vi "Check_and_rewrite_file.vi"(0 "Filename":path, 7 "Present Channels only":bool, 9 "Present Channels":string[](array[string]), 11 "Start of read offset (chars.: 0)":i32) -> (4 "exists?":bool, 6 "Merged Channels":string[](array[string]), 8 "Start of data (bytes)":i32, 10 "No of bytes/row (approx)":i32, 14 "Current file size (bytes)":i32, 15 "Merged?":bool)   [LabVIEW 2014]
uses:
  Anemometry/Anemometry Sub Vis/Globals/Constants_global.vi
panel:
  in  "stop":bool
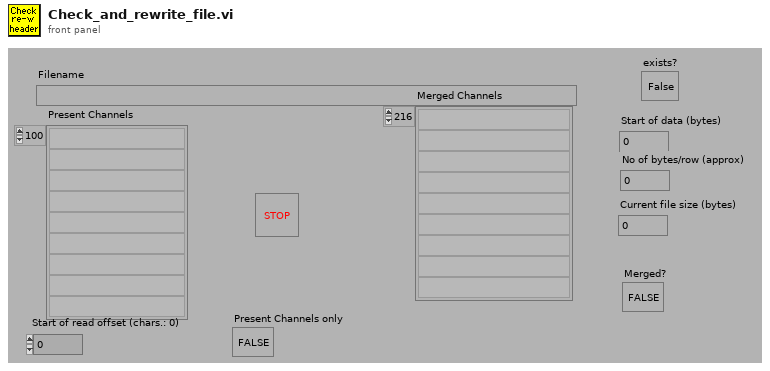
[diagram p1: front panel]
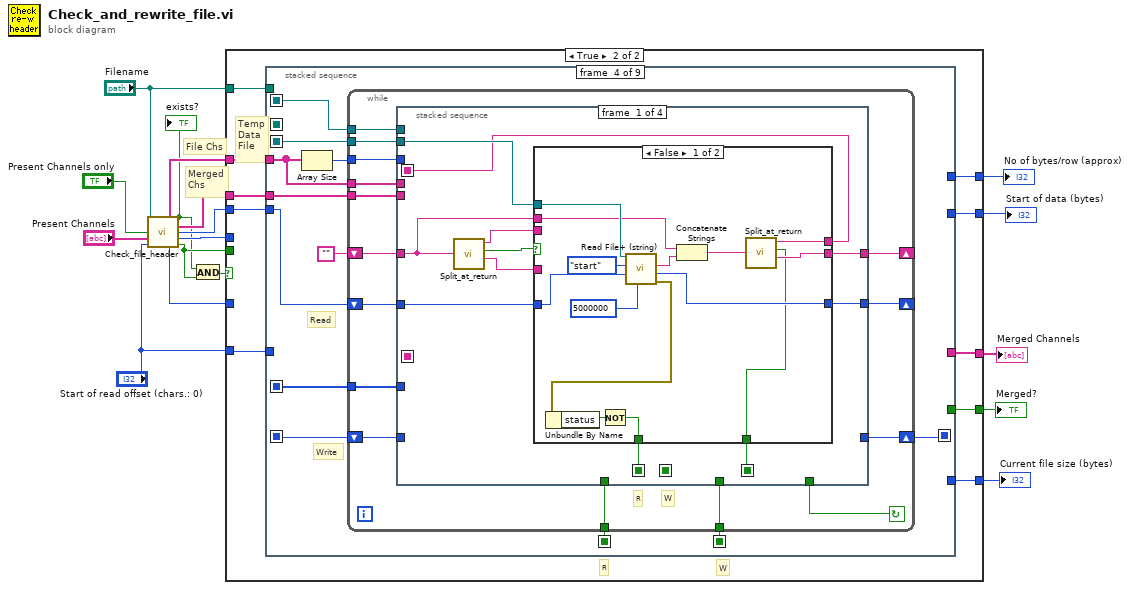
[diagram p0: block diagram]
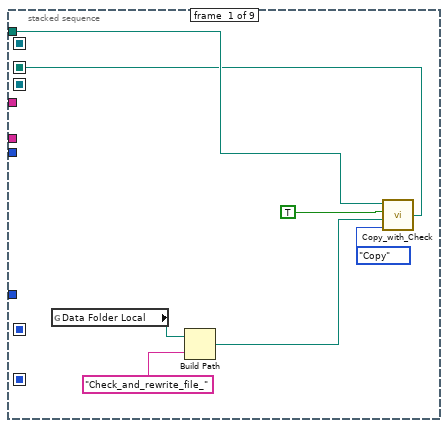
[diagram p3: hidden frame]
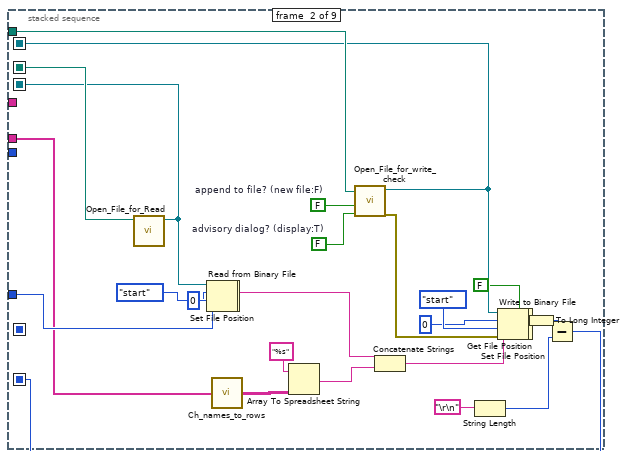
[diagram p4: hidden frame]
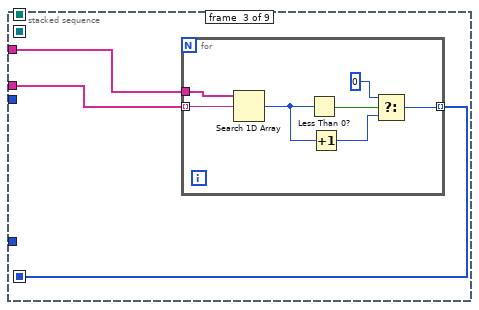
[diagram p5: hidden frame]
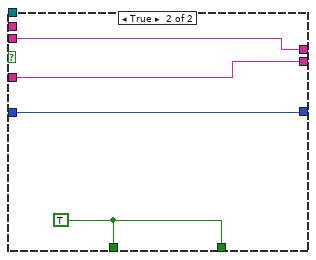
[diagram p6: hidden frame]
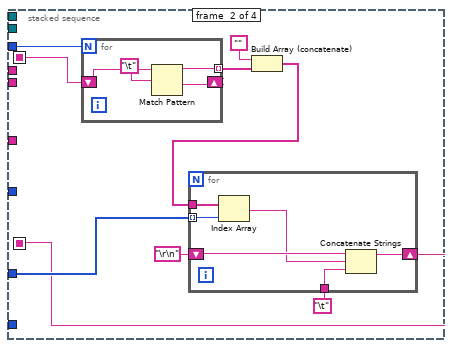
[diagram p7: hidden frame]
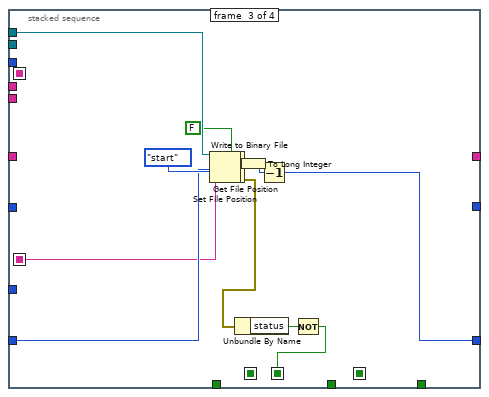
[diagram p8: hidden frame]
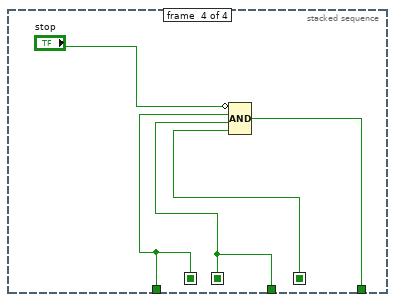
[diagram p9: hidden frame]
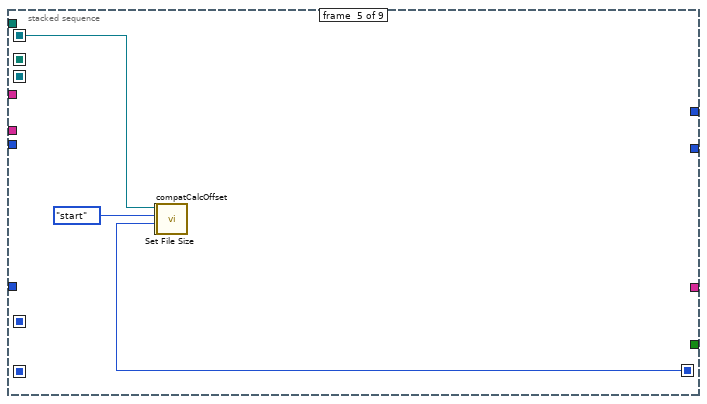
[diagram p10: hidden frame]
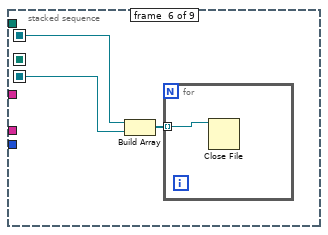
[diagram p11: hidden frame]
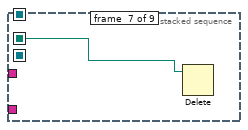
[diagram p12: hidden frame]
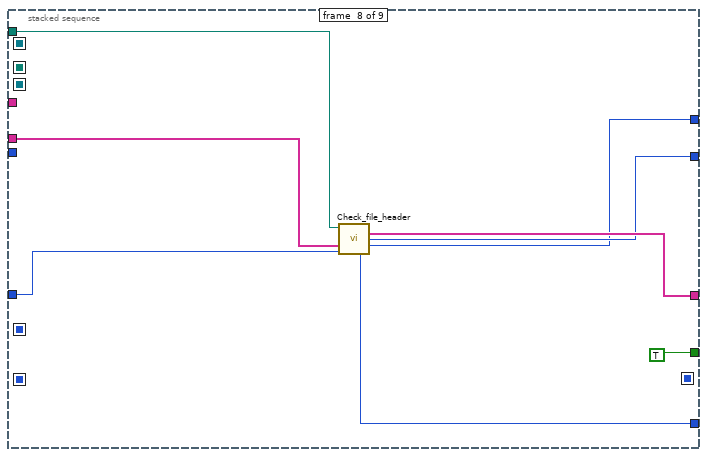
[diagram p13: hidden frame]
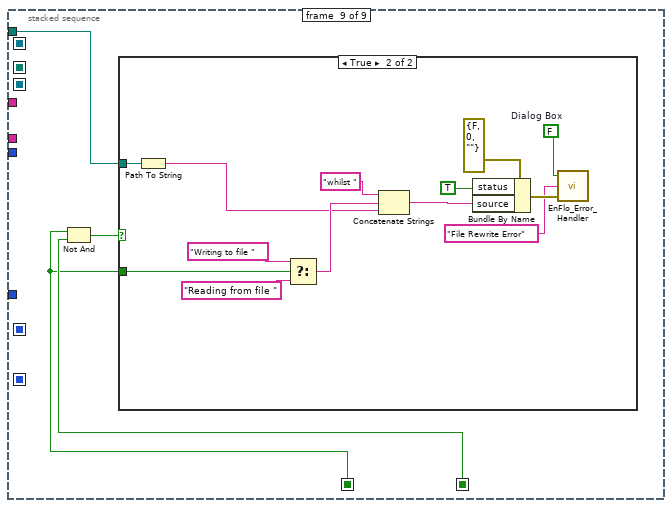
[diagram p14: hidden frame]
diagram:
  # "Merged\nChs"
  # "File Chs"
  n1 = call "Check_file_header.vi"("Filename"="Filename", "Present Channels only"="Present Channels only", "Present Channels"="Present Channels", "Start of read offset (chars.: 0)"="Start of read offset (chars.: 0)") -> ("File Channels"=w5:string[], "exists?"=w4:bool, "Merged Channels"=w11:string[], "Start of data (bytes)"=w10:i32, "No of bytes/row (approx)"=w9:i32, "Current file size (bytes)"=w8:i32, "Merged?"=w12:bool)  [unwired: 5 out]
  "exists?" <- w4
  n2 = And(x=w4, y=w12) -> (x .and. y?=w1:bool)
  n3 = case shown="True" w1 {
    tunnel: [w21 w30] -> w17
    tunnel: [w22 w29] -> w16
    tunnel: [w19 w27] -> w15
    tunnel: [w20 w28] -> w14
    tunnel: [w18 w26] -> w13
    tunnel: w12 -> [w22 _]
    tunnel: w11 -> [w21 w31]
    tunnel: w10 -> [w20 w24]
    tunnel: w9 -> [w19 _]
    tunnel: w8 -> [w18 _]
    tunnel: "Start of read offset (chars.: 0)" -> [_ w25]
    tunnel: w5 -> [_ w23]
    tunnel: "Filename" -> [_ w32]
    frame False {
    }
    frame True {
      # "W"
      # "R"
      # "Temp\nData\nFile"
      n4 = stacked-sequence {
        seq-local: [w34 _ _ _ _ _ _ _ _] -> [_ w66 _ _ _ _ w185 _ _]
        seq-local: [_ w48 _ _ _ _ _ _ _] -> [_ _ _ w90 _ w182 _ _ _]
        seq-local: [_ w65 _ _ _ _ _ _ _] -> [_ _ _ w84 w180 w183 _ _ _]
        seq-local: [_ w58 _ _ _ _ _ _ _] -> [_ _ _ w88 _ _ _ _ _]
        seq-local: [_ _ _ w83 _ _ _ _ _] -> [_ _ _ _ _ _ _ _ w195]
        seq-local: [_ _ _ w82 _ _ _ _ _] -> [_ _ _ _ _ _ _ _ w197]
        seq-local: [_ _ w70 _ _ _ _ _ _] -> [_ _ _ w81 _ _ _ _ _]
        seq-local: [_ _ _ w80 _ _ _ _ _] -> [_ _ _ _ w179 _ _ _ _]
        tunnel: w32 -> [w36 w67 _ _ _ _ _ w192 w194]
        tunnel: w31 -> [_ w50 w72 w85 _ _ _ w193 _]
        tunnel: [_ _ _ _ _ _ _ w191 _] -> w30
        tunnel: [_ _ _ _ _ _ _ TRUE _] -> w29
        tunnel: [_ _ _ _ _ _ _ w189 _] -> w28
        tunnel: [_ _ _ _ _ _ _ w188 _] -> w27
        tunnel: [_ _ _ _ _ _ _ w187 _] -> w26
        tunnel: w25 -> [_ w52 _ _ _ _ _ w186 _]
        tunnel: w24 -> [_ _ _ w89 _ _ _ _ _]
        tunnel: w23 -> [_ _ w71 w86 _ _ _ _ _]
        frame #0 {
          n5 = global read "Constants_global.vi" "Data Folder Local"() -> (w39:path)
          n6 = Build Path(base path=w39, name or relative path="Check_and_rewrite_file_") -> (appended path=w35:path)
          n7 = call "Copy_with_Check.vi"("Mode"=enum16{"Move", "Copy"}."Copy", "Target Path"=w35, "Variable Target?"=TRUE, "Source Path"=w36) -> ("Pathname Out"=w34:path)
        }
        frame #1 {
          w68 = FALSE  # advisory dialog? (display:T)
          w69 = FALSE  # append to file? (new file:F)
          n8 = call "Open_File_for_Read.vi"("file path"=w66) -> ("refnum"=w48:refnum<file>)  [unwired: 1 in, 9 out]
          n9 = Set File Position(offset (in bytes) (0)=0 ("pos offset (0)"), refnum=w48, from (0:start)=enum16{"start", "end", "current"}."start" ("pos mode (rel. to current:2)")) -> (refnum out=w47:refnum<file>, error out=w46:errorcluster)  [unwired: 1 in]
          n10 = Read from Binary File(8:w46, 10:w52, 11:w47) -> (2:w54:string)  [unwired: 6 out]
          n11 = call "Ch_names_to_rows.vi"("Channel Names"=w50) -> ("3 Row names"=w49:string[][])
          n12 = Array To Spreadsheet String(array=w49, 3:"%s" ("format string")) -> (spreadsheet string=w55:string)  [unwired: 1 out]
          n13 = call "Open_File_for_write_check.vi"("advisory dialog? (display:T)"=w68, "append to file? (new file:F)"=w69, "file path"=w67) -> ("error out"=w62:errorcluster, "refnum"=w65:refnum<file>)  [unwired: 7 out]
          n14 = Concatenate Strings(w54, w55) -> (w53:string)
          n15 = String Length(string="\r\n") -> (length=w59:i32)
          n16 = Set File Position(offset (in bytes) (0)=0 ("pos offset (0)"), refnum=w65, from (0:start)=enum16{"start", "end", "current"}."start" ("pos mode (0:2)"), error in=w62) -> (refnum out=w45:refnum<file>, error out=w44:errorcluster)
          n17 = Write to Binary File(file (use dialog)=w45, data=w53, error in=w44, 5:FALSE ("prepend array or string size? (T)")) -> (refnum out=w43:refnum<file>, error out=w42:errorcluster)  [unwired: 3 out]
          n18 = Get File Position(4:w42, 7:w43) -> (2:w41:i64)  [unwired: 2 out]
          n19 = To Long Integer(number=w41) -> (32bit integer=w60:i32)
          n20 = Subtract(x=w60, y=w59) -> (x-y=w58:i32)
        }
        frame #2 {
          n21 = for {
            tunnel: w71 -> [w79]
            tunnel: w72 -> [w78] mode=indexing
            tunnel: [w73] -> w70 mode=indexing
            n22 = Search 1D Array(1D array=w79, element=w78) -> (index of element=w76:i32)  [unwired: 1 out]
            n23 = Less Than 0?(x=w76) -> (x < 0?=w77:bool)
            n24 = Increment(x=w76) -> (x+1=w75:i32)
            n25 = Select(t=0, s=w77, f=w75) -> (s? t:f=w73:i32)
          }
        }
        frame #3 {
          # "Write"
          # "Read"
          n26 = Array Size(array=w86) -> (size(s)=w87:i32)
          n27 = while {
            tunnel: w81 -> [w92]
            tunnel: [w93] -> w82
            tunnel: [w94] -> w83
            tunnel: w84 -> [w97]
            tunnel: w85 -> [w99]
            tunnel: w86 -> [w100]
            tunnel: w87 -> [w101]
            shift-left: w88 -> [w98]
            shift-right: [w96] -> w80
            tunnel: w90 -> [w103]
            shift-left: w89 -> [w105]
            shift-right: [w104] -> _
            shift-left: "" -> [w106]
            shift-right: [w102] -> _
            stop <- w95 continue-if-true
            # "R"
            # "W"
            n28 = stacked-sequence {
              seq-local: [w109 _ _ _] -> [_ w143 _ _]
              seq-local: [_ w136 _ _] -> [_ _ w164 _]
              seq-local: [_ _ w161 _] -> [_ _ _ w170]
              seq-local: [w110 _ _ _] -> [_ _ _ w172]
              seq-local: [w111 _ _ _] -> [_ _ _ w171]
              tunnel: w106 -> [w114 _ _ _]
              tunnel: w105 -> [w117 _ _ _]
              tunnel: [w116 _ _ _] -> w104
              tunnel: w103 -> [w115 _ _ _]
              tunnel: [w113 _ _ _] -> w102
              tunnel: w101 -> [_ w144 _ _]
              tunnel: w100 -> [_ _ _ _]
              tunnel: w99 -> [_ _ _ _]
              tunnel: w98 -> [_ _ w168 _]
              tunnel: w97 -> [_ _ w167 _]
              tunnel: [_ _ w165 _] -> w96
              tunnel: [_ _ _ w173] -> w95
              tunnel: [_ _ _ w171] -> w94
              tunnel: [_ _ _ w170] -> w93
              tunnel: w92 -> [_ w139 _ _]
              frame #0 {
                n29 = call "Split_at_return.vi"("String"=w114) -> ("before substring"=w108:string, "Matched?"=w107:bool, "after substring"=w112:string)  [unwired: 1 in, 1 out]
                n30 = case shown="False" w107 {
                  tunnel: w117 -> [w131 w135]
                  tunnel: [w129 w135] -> w116
                  tunnel: w115 -> [w128 _]
                  tunnel: w114 -> [w126 _]
                  tunnel: [w124 w134] -> w113
                  tunnel: w112 -> [_ w134]
                  tunnel: [w121 w133] -> w111
                  tunnel: [w119 w133] -> w110
                  tunnel: [w120 w132] -> w109
                  tunnel: w108 -> [_ w132]
                  frame False {
                    n31 = call <vilib>:"Read File+ (string).vi"("count"=5000000, "pos offset (bytes:0)"=w131, "pos mode (rel. to current:2)"=enum16{"start", "end", "current"}."start", "refnum"=w128) -> ("error out"=w123:errorcluster, "mark after read (bytes)"=w129:i32, "string"=w127:string)  [unwired: 1 in, 4 out]
                    n32 = Unbundle By Name(w123) -> ("status"=w122:bool)
                    n33 = Not(x=w122) -> (.not. x?=w121:bool)
                    n34 = Concatenate Strings(w126, w127) -> (w125:string)
                    n35 = call "Split_at_return.vi"("String"=w125) -> ("before substring"=w120:string, "Matched?"=w119:bool, "after substring"=w124:string)  [unwired: 1 in, 1 out]
                  }
                  frame True {
                    w133 = TRUE
                  }
                }
              }
              frame #1 {
                n36 = for {
                  N: w144 -> [_]
                  shift-right: [w152] -> _
                  shift-left: w143 -> [w153]
                  tunnel: [w151] -> w141 mode=indexing
                  n37 = Match Pattern(string=w153, regular expression="\t") -> (before substring=w151:string, after substring=w152:string)  [unwired: 3 out]
                }
                n38 = Build Array (concatenate)("", w141) -> (w140:string[])
                n39 = for {
                  tunnel: w139 -> [w150] mode=indexing
                  tunnel: w140 -> [w149]
                  shift-right: [w145] -> w136
                  shift-left: "\r\n" -> [w148]
                  tunnel: "\t" -> [w146]
                  n40 = Index Array(array=w149, index=w150) -> (element=w147:string)
                  n41 = Concatenate Strings(w148, w147, w146) -> (w145:string)
                }
              }
              frame #2 {
                n42 = Set File Position(offset (in bytes) (0)=w168, refnum=w167, from (0:start)=enum16{"start", "end", "current"}."start" ("pos mode (0:2)")) -> (refnum out=w160:refnum<file>, error out=w159:errorcluster)  [unwired: 1 in]
                n43 = Write to Binary File(file (use dialog)=w160, data=w164, error in=w159, 5:FALSE ("prepend array or string size? (T)")) -> (refnum out=w158:refnum<file>, error out=w157:errorcluster)  [unwired: 3 out]
                n44 = Get File Position(4:w157, 7:w158) -> (0:w163:errorcluster, 2:w156:i64)  [unwired: 1 out]
                n45 = Unbundle By Name(w163) -> ("status"=w162:bool)
                n46 = To Long Integer(number=w156) -> (32bit integer=w166:i32)
                n47 = Decrement(x=w166) -> (x-1=w165:i32)
                n48 = Not(x=w162) -> (.not. x?=w161:bool)
              }
              frame #3 {
                n49 = Compound Arithmetic op=AND(invert "stop", w171, w170, w172) -> (w173:bool)
              }
            }
          }
        }
        frame #4 {
          n50 = call <vilib>:"compatCalcOffset.vi"("pos offset (0)"=w179, "pos mode (0:1)"=enum16{"start", "end", "current"}."start", "refnum"=w180) -> ("error out"=w177:errorcluster, "offset"=w176:i32, "dup refnum"=w175:refnum<file>)  [unwired: 1 in, 5 out]
          n51 = Set File Size(4:w177, 6:w176, 7:w175) -> ()  [unwired: 2 out]
        }
        frame #5 {
          n52 = Build Array(w183, w182) -> (w181:refnum<file>[])
          n53 = for {
            tunnel: w181 -> [w184] mode=indexing
            n54 = Close File(refnum=w184) -> ()  [unwired: 1 in, 2 out]
          }
        }
        frame #6 {
          n55 = Delete(path (use dialog)=w185) -> ()  [unwired: 1 in, 6 out]
        }
        frame #7 {
          n56 = call "Check_file_header.vi"("Filename"=w192, "Present Channels"=w193, "Start of read offset (chars.: 0)"=w186) -> ("Merged Channels"=w191:string[], "Start of data (bytes)"=w189:i32, "No of bytes/row (approx)"=w188:i32, "Current file size (bytes)"=w187:i32)  [unwired: 1 in, 8 out]
        }
        frame #8 {
          n57 = Not And(1:w197, 2:w195) -> (0:w196:bool)
          n58 = case shown="True" w196 {
            tunnel: w195 -> [_ w210]
            tunnel: w194 -> [_ w200]
            frame False {
            }
            frame True {
              w203 = FALSE  # Dialog Box
              n59 = Path To String(path=w200) -> (string=w199:string)
              n60 = Select(t="Writing to file ", s=w210, f="Reading from file ") -> (s? t:f=w206:string)
              n61 = Concatenate Strings("whilst ", w206, w199) -> (w201:string)
              n62 = Bundle By Name(cluster=errorcluster {"status"=FALSE, "code"=0, "source"=""} ("error in (no error)"), "status"=TRUE ("Bundle Element"), "source"=w201) -> (w204:errorcluster)
              n63 = call "EnFlo_Error_Handler.vi"("error in (no error)"=w204, "Error Type"="File Rewrite Error", "Dialog Box (T)"=w203) -> ()  [unwired: 3 out]
            }
          }
        }
      }
    }
  }
  "Merged?" <- w16
  "Merged Channels" <- w17
  "Current file size (bytes)" <- w13
  "Start of data (bytes)" <- w14
  "No of bytes/row (approx)" <- w15
